vi "CLD 6 CSV file utility Solution.vi"(8 "Fehler (Eingang)":T1, 10 "[Daten, Eingang]":T2[](array[typedef]), 11 "CSV lesen/CSV schreiben":T3) -> (0 "Fehler (Ausgang)":T1, 3 "[Daten, Ausgang]":T2[](array[typedef]))   [LabVIEW 2009]
doc: "CLD 6\n\nDieses VI ist ein Hilfs-VI zum Auslesen der Datei \"CLD CSV File.csv\" und Einfügen der Daten in den Daten-Cluster \"CLD Six CSV file data structure.ctl\".\n\nHinweis für das Testen:\n\nEs ist ein boolesches Element vorhanden, mit dem sichergestellt werden kann, dass die FGV entweder im gleichen Verzeichnis, in dem sich auch die FGV befindet (nützlich für das Testen), oder im Verzeichnis des Aufrufers nach der Datendatei sucht, wenn sich der Aufrufer in einer Standard-CLD-Testhierarchie eine Verzeichnisebene über dem SubVI-Verzeichnis befindet."
uses:
  CLD 6 CSV file data structure.ctl
  <vilib>/Utility/file.llb/Write To Spreadsheet File (string).vi
  <vilib>/Utility/file.llb/Read From Spreadsheet File (string).vi
  CLD 6 CSV file enum.ctl
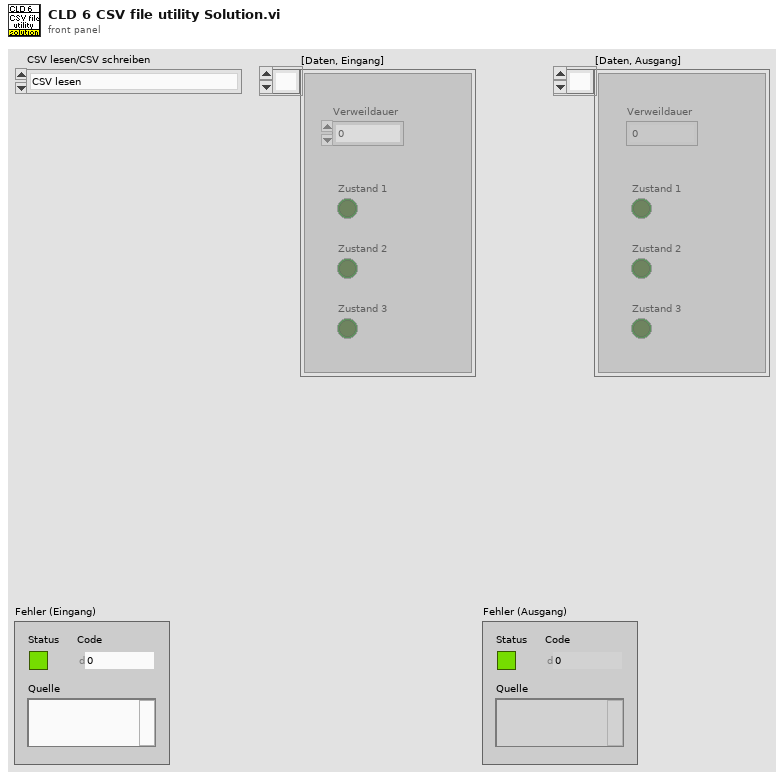
[diagram p1: front panel]
types:
  T1 = cluster{"Status":bool, "Code":i32, "Quelle":string}
  T2 = typedef "CLD 6 CSV file data structure.ctl" = cluster{"Verweildauer":i32, "Zustand 1":bool, "Zustand 2":bool, "Zustand 3":bool}
  T3 = typedef "CLD 6 CSV file enum.ctl" = enum16{"CSV lesen", "CSV schreiben"}
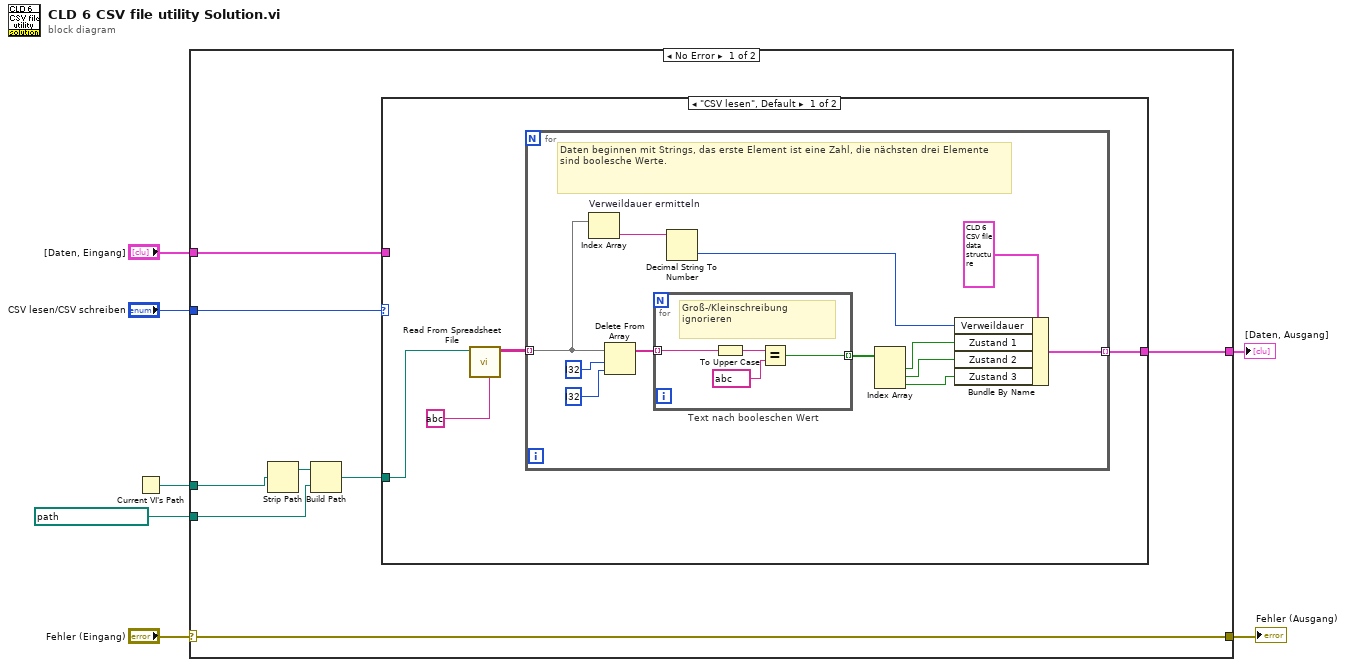
[diagram p0: block diagram]
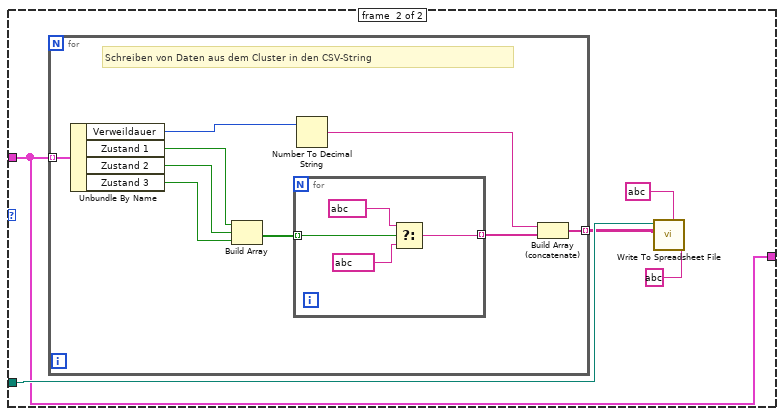
[diagram p2: hidden frame]
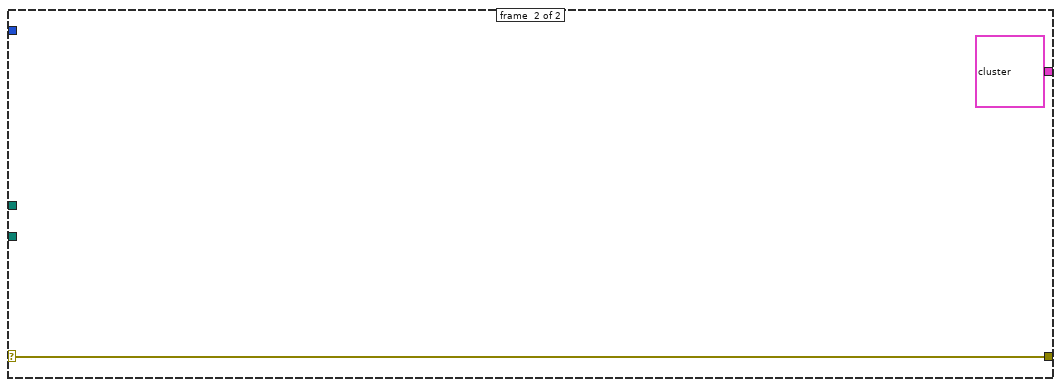
[diagram p3: hidden frame]
diagram:
  n1 = Current VI's Path() -> (path=w5:path)
  n2 = case shown="No Error" "Fehler (Eingang)" {
    selector: "Fehler (Eingang)" -> [w9 w55]
    tunnel: [w15 T2[] ? ("[Daten, Eingang]")] -> w7
    tunnel: path ? -> [w14 _]
    tunnel: w5 -> [w13 _]
    tunnel: "CSV lesen/CSV schreiben" -> [w11 _]
    tunnel: "[Daten, Eingang]" -> [w10 _]
    tunnel: [w9 w55] -> w1
    frame #0 {
      n3 = Strip Path(path=w13) -> (stripped path=w8:path)  [unwired: 1 out]
      n4 = Build Path(base path=w8, name or relative path=w14) -> (appended path=w12:path)
      n5 = case shown="\"CSV lesen\", Default" w11 {
        tunnel: w12 -> [w19 w40]
        tunnel: [w17 w36] -> w15
        tunnel: w10 -> [_ w36]
        frame #0 {
          n6 = call-poly <vilib>:"Read From Spreadsheet File.vi"("delimiter (\\t)"=string ? ("Trennzeichen (\\t)"), "file path (dialog if empty)"=w19) -> ("all rows"=w18:string[][])  [unwired: 5 in, 4 out]
          n7 = for {
            tunnel: w18 -> [w28] mode=indexing
            tunnel: [w31] -> w17 mode=indexing
            # "Daten beginnen mit Strings, das erste Element ist eine Zahl, die nächsten drei Elemente sind boolesche Werte."
            n8 = Index Array "Verweildauer ermitteln"(array=w28) -> (element=w30:string)  [unwired: 1 in]
            n9 = Delete From Array(array=w28, length=i32 ? ("Länge"), index=i32 ? ("Index")) -> (array with subset deleted=w21:string[])  [unwired: 1 out]
            n10 = for "Text nach booleschen Wert" {
              tunnel: w21 -> [w35] mode=indexing
              tunnel: [w32] -> w25 mode=indexing
              # "Groß-/Kleinschreibung ignorieren"
              n11 = To Upper Case(1:w35) -> (0:w34:string)
              n12 = Equal?(x=w34, y=string ?) -> (x = y?=w32:bool)
            }
            n13 = Decimal String To Number(string=w30) -> (number=w29:i32)  [unwired: 2 in, 1 out]
            n14 = Index Array(array=w25) -> (element #1=w24:bool, element #2=w23:bool, element #3=w22:bool)  [unwired: 3 in]
            n15 = Bundle By Name(cluster=T2 ? ("Datenstruktur der CSV-Datei"), "Verweildauer"=w29, "Zustand 1"=w24, "Zustand 2"=w23, "Zustand 3"=w22) -> (w31:T2)
          }
        }
        frame #1 {
          n16 = for {
            tunnel: w36 -> [w49] mode=indexing
            tunnel: [w41] -> w38 mode=indexing
            # "Schreiben von Daten aus dem Cluster in den CSV-String"
            n17 = Unbundle By Name(w49) -> ("Verweildauer"=w48:i32, "Zustand 1"=w47:bool, "Zustand 2"=w46:bool, "Zustand 3"=w45:bool)
            n18 = Build Array(w47, w46, w45) -> (w44:bool[])
            n19 = for {
              tunnel: w44 -> [w53] mode=indexing
              tunnel: [w50] -> w42 mode=indexing
              n20 = Select(t=string ?, s=w53, f=string ?) -> (s? t:f=w50:string)
            }
            n21 = Number To Decimal String(number=w48) -> (decimal integer string=w43:string)  [unwired: 1 in]
            n22 = Build Array (concatenate)(w43, w42) -> (w41:string[])
          }
          n23 = call-poly <vilib>:"Write To Spreadsheet File.vi"("delimiter (\\t)"=string ? ("Trennzeichen (\\t)"), "format (%s)"=string ? ("Format (%s)"), "2D data"=w38, "file path (dialog if empty)"=w40) -> ()  [unwired: 4 in, 1 out]
        }
      }
    }
    frame #1 {
    }
  }
  "[Daten, Ausgang]" <- w7
  "Fehler (Ausgang)" <- w1
